vi "Get Analog Channel State.vi"(8 "error in (no error)":errorcluster, 10 "Analog Channel":T1, 11 "DPO4104 in":refnum<class "DPO4104.lvclass">) -> (0 "error out":errorcluster, 2 "Channel State (T = ON)":bool, 3 "DPO4104 out":refnum<class "DPO4104.lvclass">)   [LabVIEW 2018, in "DPO4104.lvlib" / "DPO4104.lvclass"]
doc: "This method gets the state (T=ON, F=OFF) for the selected channel."
uses:
  DPO4104.lvclass
  PPLs/Oscilloscope/Parent/Oscilloscope.lvlibp/Custom Controls/Analog Channels.ctl
  PPLs/Oscilloscope/Parent/Oscilloscope.lvlibp/Oscilloscope.lvclass
  C:/Projects/LabVIEW/PPLs/Oscilloscope/Parent/Oscilloscope.lvlibp/Oscilloscope.lvclass
  PPLs/Oscilloscope/Parent/Oscilloscope.lvlibp
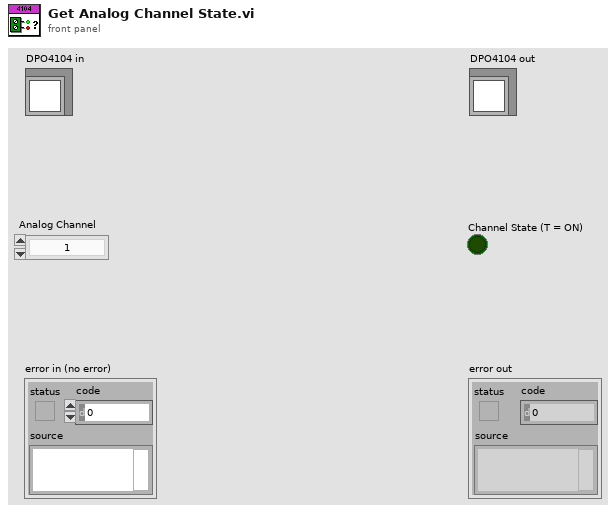
[diagram p1: front panel]
types:
  T1 = typedef "Oscilloscope.lvlibp/Analog Channels.ctl" = enum16{"1", "2", "3", "4", "5", "6", "7", "8", "9", "10", "11", "12", "13", "14", "15", "16"}
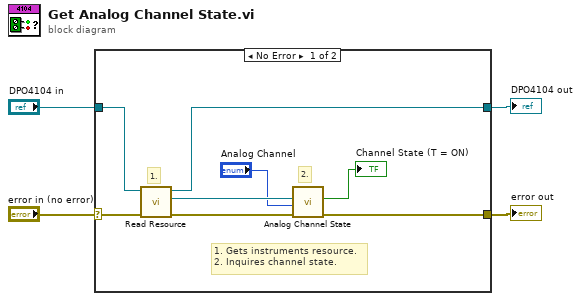
[diagram p0: block diagram]
diagram:
  n1 = case shown="No Error" "error in (no error)" {
    selector: "error in (no error)" -> [w10 w14]
    tunnel: [w7 w14] -> w3
    tunnel: [w11 w13] -> w1
    tunnel: "DPO4104 in" -> [w12 w13]
    frame No Error {
      # "2."
      # "1."
      # "1. Gets instruments resource.\n2. Inquires channel state."
      n2 = call "Read Resource.vi"("error in (no error)"=w10, "Oscilloscope in"=w12) -> ("error out"=w8:errorcluster, "Resource"=w9:refnum<visa-resource-name>, "Oscilloscope out"=w11:refnum<class "DPO4104.lvclass">)  [unwired: 7 in]
      n3 = call "Analog Channel State.vi"("error in (no error)"=w8, "Analog Channel"="Analog Channel", "VISA resource name"=w9) -> ("error out"=w7:errorcluster, "Channel State (T = ON)"=→"Channel State (T = ON)":bool)  [unwired: 6 in, 1 out]
    }
    frame Error {
    }
  }
  "error out" <- w3
  "DPO4104 out" <- w1
